vi "WPI_CameraGet Image From TCP.vi"(8 "error in (no error)":errorcluster, 9 "Unflatten":bool, 10 "Image In":T1, 11 "connection ID":refnum<k5>) -> (0 "error out":errorcluster, 1 "Size":i32, 2 "Image Out":T1, 3 "connection ID (dup)":refnum<k5>)   [LabVIEW 2017]
doc: "This software is licensed. Open the labview\\readme\\WPI Robotics Library Open Source License.txt file for more information."
uses:
  <vilib>/vision/Image Controls.llb/IMAQ Image.ctl
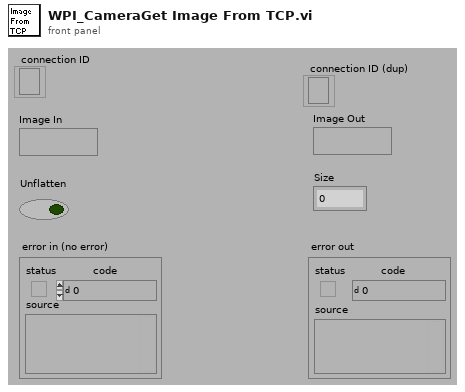
[diagram p1: front panel]
types:
  T1 = typedef "IMAQ Image.ctl" = refnum<image>
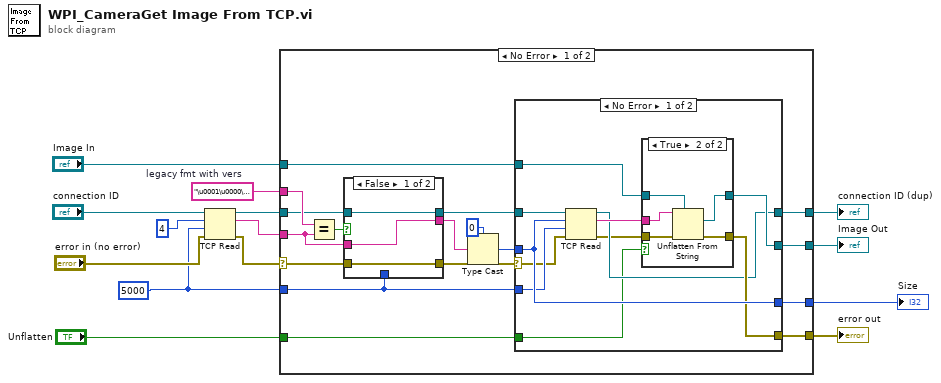
[diagram p0: block diagram]
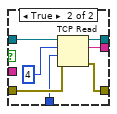
[diagram p2: hidden frame]
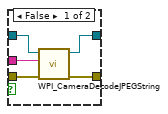
[diagram p3: hidden frame]
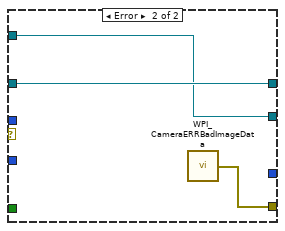
[diagram p4: hidden frame]
diagram:
  w2 = 5000 ("bytes to read")
  w3 = "\u0001\u0000\u0000\u0000"  # legacy fmt with vers
  n1 = TCP Read(connection ID="connection ID", bytes to read=4, error in (no error)="error in (no error)", 9:w2) -> (connection ID out=w14:refnum<k5>, data out=w10:string, error out=w5:errorcluster)  [unwired: 1 out]
  n2 = case shown="No Error" w5 {
    selector: w5 -> [w23 w66]
    tunnel: w14 -> [w25 w68]
    tunnel: "Image In" -> [w31 w67]
    tunnel: w10 -> [w22 _]
    tunnel: [w30 w66] -> w8
    tunnel: [w29 w67] -> w7
    tunnel: [w28 w68] -> w6
    tunnel: [w27 _] -> w4
    tunnel: w3 -> [w26 _]
    tunnel: "Unflatten" -> [w15 _]
    tunnel: w2 -> [w16 _]
    frame No Error {
      n3 = Equal?(x=w26, y=w22) -> (x = y?=w20:bool)
      n4 = case shown="False" w20 {
        tunnel: w25 -> [w34 w40]
        tunnel: [w34 w39] -> w24
        tunnel: w23 -> [w33 w38]
        tunnel: [w33 w37] -> w18
        tunnel: [w32 w36] -> w19
        tunnel: w22 -> [w32 _]
        tunnel: w16 -> [_ w35]
        frame False {
        }
        frame True {
          n5 = TCP Read(connection ID=w40, bytes to read=4, error in (no error)=w38, 9:w35) -> (connection ID out=w39:refnum<k5>, data out=w36:string, error out=w37:errorcluster)  [unwired: 1 out]
        }
      }
      n6 = Type Cast(type=0 ("bytes to read"), x=w19) -> (*(type *) &x=w17:i32)
      n7 = case shown="No Error" w18 {
        selector: w18 -> [w47 _]
        tunnel: w24 -> [w52 w65]
        tunnel: w31 -> [w49 w64]
        tunnel: [w46 w63] -> w30
        tunnel: [w48 w64] -> w29
        tunnel: [w44 w65] -> w28
        tunnel: [w51 _] -> w27
        tunnel: w17 -> [w51 _]
        tunnel: w16 -> [w50 _]
        tunnel: w15 -> [w43 _]
        frame No Error {
          n8 = TCP Read(connection ID=w52, bytes to read=w51, error in (no error)=w47, 9:w50) -> (connection ID out=w44:refnum<k5>, data out=w45:string, error out=w42:errorcluster)  [unwired: 1 out]
          n9 = case shown="True" w43 {
            tunnel: w49 -> [w57 w61]
            tunnel: [w56 w62] -> w48
            tunnel: w45 -> [w55 w59]
            tunnel: [w54 w60] -> w46
            tunnel: w42 -> [w53 w58]
            frame False {
              n10 = call <vilib>:"WPI_CameraDecodeJPEGString.vi"("error in"=w53, "Compressed Image"=w55, "Image In"=w57) -> ("error out"=w54:errorcluster, "Image Out"=w56:T1)  [unwired: 3 out]
            }
            frame True {
              n11 = Unflatten From String(type=w61, binary string=w59, error in (no error)=w58) -> (value=w62:T1, error out=w60:errorcluster)  [unwired: 2 in, 1 out]
            }
          }
        }
        frame Error {
          n12 = call <vilib>:"WPI_CameraERRBadImageData.vi"() -> ("error out"=w63:errorcluster)
        }
      }
    }
    frame Error {
    }
  }
  "error out" <- w8
  "Image Out" <- w7
  "connection ID (dup)" <- w6
  "Size" <- w4
